vi "维持时间.vi"(8 "错误输入":errorcluster, 10 "参数":T1, 11 "VISA资源名称":refnum<visa-resource-name>) -> (0 "错误输出":errorcluster, 3 "VISA资源名称输出":refnum<visa-resource-name>)   [LabVIEW 2019]
uses:
  lib/Global variable.vi
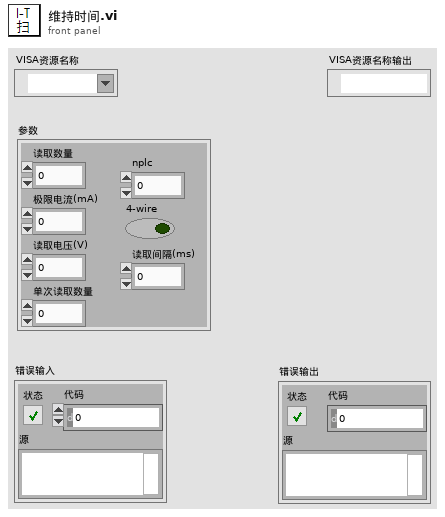
[diagram p1: front panel]
types:
  T1 = cluster{"nplc":dbl, "4-wire":bool, "读取间隔(ms)":dbl, "读取数量":dbl, "极限电流(mA)":dbl, "读取电压(V)":dbl, "单次读取数量":dbl}
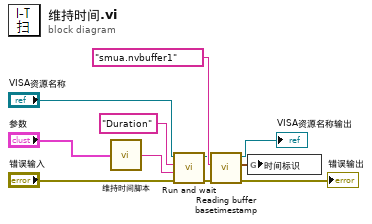
[diagram p0: block diagram]
diagram:
  n1 = call "维持时间脚本.vi"("参数"="参数") -> ("Script"=w1:string)
  n2 = call "Run and wait.vi"("错误输入"="错误输入", "Script"=w1, "Script Name"="Duration", "VISA资源名称"="VISA资源名称") -> ("错误输出"=w8:errorcluster, "VISA资源名称输出"=w9:refnum<visa-resource-name>)  [unwired: 6 in]
  n3 = call "Reading buffer basetimestamp.vi"("错误输入"=w8, "缓冲区名称"="smua.nvbuffer1", "VISA资源名称"=w9) -> ("错误输出"=→"错误输出":errorcluster, "时间标识"=w11:timestamp, "VISA资源名称输出"=→"VISA资源名称输出":refnum<visa-resource-name>)  [unwired: 6 in]
  n4 = global write "Global variable.vi" "时间标识"(w11) -> ()
